vi "Read Named ROI.vi"(8 "error in (no error)":errorcluster, 11 "ROI Name Dialog in":refnum<class "ROI Name Dialog.lvclass">) -> (0 "error out":errorcluster, 2 "Named ROI":T1, 3 "ROI Name Dialog out":refnum<class "ROI Name Dialog.lvclass">)   [LabVIEW 2014, in "ROI Name Dialog.lvlib" / "ROI Name Dialog.lvclass"]
uses:
  ROI Name Dialog.lvclass
  HIJ Vision Display/HIJ Vision Display/Named ROI.ctl
  ROI Name Dialog.lvclass/ROI Name Dialog.ctl
  HIJ Vision Display/HIJ Vision Display/HIJ Vision Display.lvclass
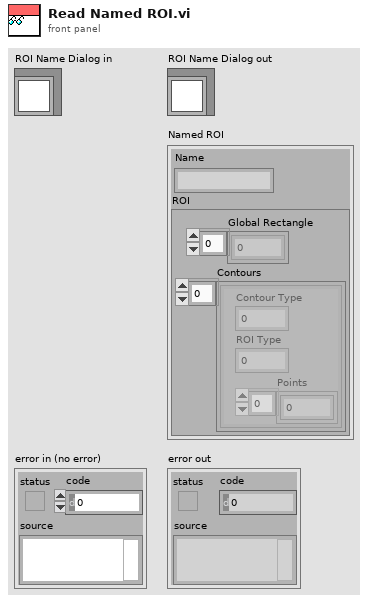
[diagram p1: front panel]
types:
  T1 = typedef "HIJ Vision Display.lvlib/HIJ Vision Display.lvclass/Named ROI.ctl" = cluster{"ROI":cluster{"Global Rectangle":i32[], "Contours":cluster{"Contour Type":u32, "ROI Type":u32, "Points":i32[]}[]}, "Name":string}
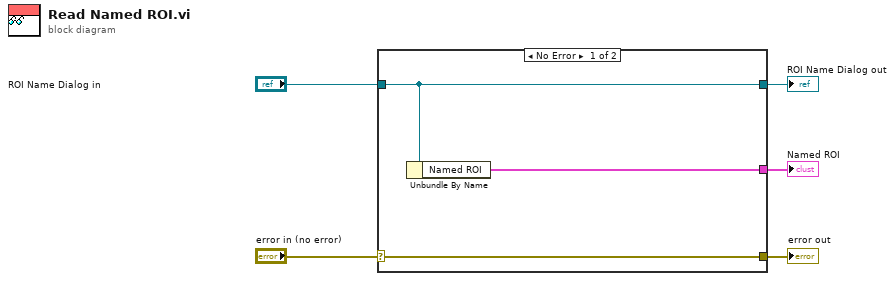
[diagram p0: block diagram]
diagram:
  n1 = case shown="No Error" "error in (no error)" {
    selector: "error in (no error)" -> [w8 w9]
    tunnel: [w8 w9] -> w4
    tunnel: [w7 w10] -> w2
    tunnel: "ROI Name Dialog in" -> [w7 w10]
    tunnel: [w6 _] -> w1
    frame No Error {
      n2 = Unbundle By Name(w7) -> ("Named ROI"=w6:T1)
    }
    frame Error {
    }
  }
  "error out" <- w4
  "ROI Name Dialog out" <- w2
  "Named ROI" <- w1
